vi "Write Element of Timeouts.vi"(8 "error in (no error)":errorcluster, 9 "Timeout":refnum<class "Timeout.lvclass">, 10 "index":i32, 11 "State in":refnum<class "State.lvclass">) -> (0 "error out":errorcluster, 3 "State out":refnum<class "State.lvclass">)   [LabVIEW 2020, in "State.lvclass"]
uses:
  State.lvclass
  Timeout/Timeout.lvclass
  State.lvclass/State.ctl
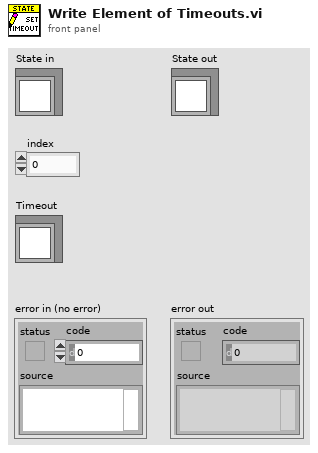
[diagram p1: front panel]
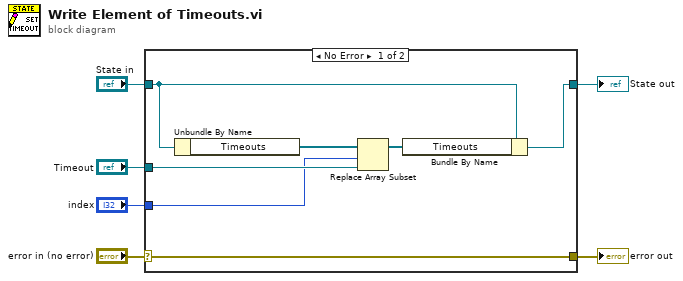
[diagram p0: block diagram]
diagram:
  n1 = case shown="No Error" "error in (no error)" {
    selector: "error in (no error)" -> [w13 w14]
    tunnel: [w13 w14] -> w5
    tunnel: [w12 w15] -> w3
    tunnel: "State in" -> [w11 w15]
    tunnel: "Timeout" -> [w8 _]
    tunnel: "index" -> [w7 _]
    frame No Error {
      n2 = Unbundle By Name(w11) -> ("Timeouts"=w10:refnum<class "Timeout.lvclass">[])
      n3 = Replace Array Subset(array=w10, new element=w8, index=w7) -> (w9:refnum<class "Timeout.lvclass">[])
      n4 = Bundle By Name(cluster=w11, "Timeouts"=w9) -> (w12:refnum<class "State.lvclass">)
    }
    frame Error {
    }
  }
  "error out" <- w5
  "State out" <- w3
